vi "From Serial Form.vi"(6 "Serial Version":T1, 10 "Deserializer in":refnum<class "Deserializer.lvclass">, 11 "PAS Cell Data in":refnum<class "PAS Cell Data.lvclass">) -> (0 "error out":errorcluster, 2 "Deserializer out":refnum<class "Deserializer.lvclass">, 3 "PAS Cell Data out":refnum<class "PAS Cell Data.lvclass">)   [LabVIEW 2014, in "PAS Cell Data.lvclass"]
uses:
  PAS Cell Data.lvclass
  <vilib>/NI/AQ Character Lineator/Deserializer/Deserializer.lvclass
  <vilib>/NI/AQ Character Lineator/Serialization Common/Serial Version.ctl
  PAS Cell Data.lvclass/PAS Cell Data.ctl
  <vilib>/NI/AQ Character Lineator/Serializable/Remove Double Array.vi
  <vilib>/NI/AQ Character Lineator/Serializable/Remove Double.vi
  <vilib>/Analysis/Matrix/Numeric/Conversions/Array To Matrix - RA2.vi
  Data/Data.lvclass
  <vilib>/NI/AQ Character Lineator/Serializable/Serializable.lvclass
  <vilib>/Analysis/Matrix/NI_Matrix.lvlib
  <vilib>/NI/AQ Character Lineator/Serializable Analog Waveform/Serializable Analog Waveform.lvclass
  <vilib>/NI/AQ Character Lineator/Serialization Common/Serialization Common.lvlib
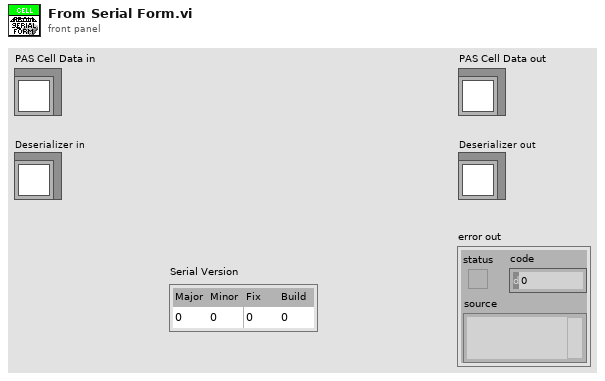
[diagram p1: front panel]
types:
  T1 = typedef "Serialization Common.lvlib/Serial Version.ctl" = cluster{"Major":u16, "Minor":u16, "Fix":u16, "Build":u16}
  T2 = typedef "NI_Matrix.lvlib/RealMatrix.ctl" = dbl[][]
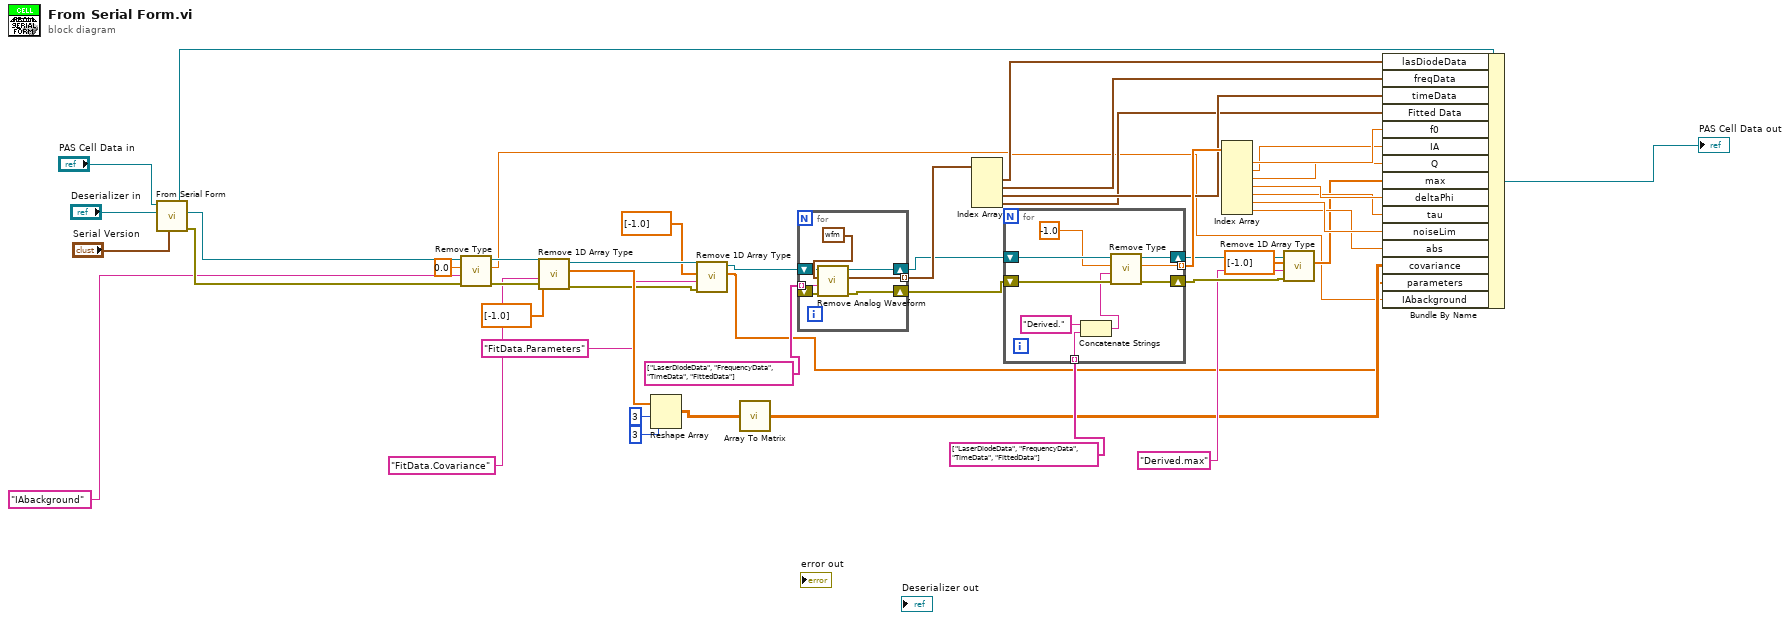
[diagram p0: block diagram]
diagram:
  n1 = call-parent "From Serial Form.vi"("Serial Version"="Serial Version", "Deserializer in"="Deserializer in", "Data in"="PAS Cell Data in") -> ("error out"=w43:errorcluster, "Deserializer out"=w44:refnum<class "Deserializer.lvclass">, "Data out"=w18:refnum<class "PAS Cell Data.lvclass">)  [unwired: 6 in]
  n2 = call-poly <vilib>:"Remove Type.vi"("error in (no error)"=w43, "Name"="IAbackground", "Default Value"=0.0, "Deserializer in"=w44) -> ("error out"=w39:errorcluster, "Numeric"=w2:dbl, "Deserializer out"=w40:refnum<class "Deserializer.lvclass">)  [unwired: 4 in, 1 out]
  n3 = call-poly <vilib>:"Remove 1D Array Type.vi"("error in (no error)"=w39, "Name"="FitData.Covariance", "Default Value"=dbl[] [-1.0], "Deserializer in"=w40) -> ("error out"=w32:errorcluster, "Doubles"=w34:dbl[], "Deserializer out"=w33:refnum<class "Deserializer.lvclass">)  [unwired: 4 in, 1 out]
  n4 = Reshape Array(w34, 3 ("dimension size"), 3 ("dimension size")) -> (w35:dbl[][])
  n5 = call-poly <vilib>:"Remove 1D Array Type.vi"("error in (no error)"=w32, "Name"="FitData.Parameters", "Default Value"=dbl[] [-1.0], "Deserializer in"=w33) -> ("Doubles"=w3:dbl[], "Deserializer out"=w28:refnum<class "Deserializer.lvclass">)  [unwired: 4 in, 2 out]
  n6 = call-poly <vilib>:"Array To Matrix.vi"("Real 2D Array"=w35) -> ("Real Matrix"=w4:T2)
  n7 = for {
    tunnel: string[] ["LaserDiodeData", "FrequencyData", "TimeData", "FittedData"] -> [w53] mode=indexing
    shift-right: [w51] -> w26
    shift-left: w28 -> [w52]
    shift-right: [w50] -> w25
    shift-left: _ -> [w49]
    tunnel: [w48] -> w27 mode=indexing
    n8 = call <vilib>:"Remove Analog Waveform.vi"("error in (no error)"=w49, "Name"=w53, "Default Value"=waveform(dbl) {"t0"=timestamp(0 s since 1904-01-01), "dt"=1.0, "Y"=[]}, "Deserializer in"=w52) -> ("error out"=w50:errorcluster, "Analog Waveform"=w48:waveform(dbl), "Deserializer out"=w51:refnum<class "Deserializer.lvclass">)  [unwired: 4 in, 1 out]
  }
  n9 = Index Array(array=w27) -> (element #1=w9:waveform(dbl), element #2=w8:waveform(dbl), element #3=w7:waveform(dbl), element #4=w6:waveform(dbl))  [unwired: 4 in]
  n10 = for {
    shift-right: [w60] -> w21
    shift-left: w25 -> [w62]
    shift-right: [w61] -> w22
    shift-left: w26 -> [w63]
    tunnel: string[] ["LaserDiodeData", "FrequencyData", "TimeData", "FittedData"] -> [w57] mode=indexing
    tunnel: [w55] -> w23 mode=indexing
    n11 = Concatenate Strings("Derived." ("string"), w57) -> (w58:string)
    n12 = call-poly <vilib>:"Remove Type.vi"("error in (no error)"=w62, "Name"=w58, "Default Value"=-1.0, "Deserializer in"=w63) -> ("error out"=w60:errorcluster, "Numeric"=w55:dbl, "Deserializer out"=w61:refnum<class "Deserializer.lvclass">)  [unwired: 4 in, 1 out]
  }
  n13 = Index Array(array=w23) -> (element #1=w17:dbl, element #2=w16:dbl, element #3=w15:dbl, element #4=w14:dbl, element #5=w13:dbl, element #6=w12:dbl, element #7=w11:dbl)  [unwired: 7 in]
  n14 = call-poly <vilib>:"Remove 1D Array Type.vi"("error in (no error)"=w21, "Name"="Derived.max", "Default Value"=dbl[] [-1.0], "Deserializer in"=w22) -> ("Doubles"=w10:dbl[])  [unwired: 4 in, 3 out]
  n15 = Bundle By Name(cluster=w18, "lasDiodeData"=w9, "freqData"=w8, "timeData"=w7, "Fitted Data"=w6, "f0"=w17, "IA"=w16, "Q"=w15, "max"=w10, "deltaPhi"=w14, "tau"=w13, "noiseLim"=w12, "abs"=w11, "covariance"=w4, "parameters"=w3, "IAbackground"=w2) -> (→"PAS Cell Data out":refnum<class "PAS Cell Data.lvclass">)
